vi "Update All Timestamps.vi"(10 "New offset (ns)":i64, 11 "Bytes in":u8[](array[numeric])) -> (2 "Records":i32, 3 "Bytes out":u8[](array[numeric]))   [LabVIEW 2021, in "pcap_Parse_Build_CIF.lvclass"]
doc: "Update all timestamps in the pcap bytestream. This will automatically detect if a global header is present and will work on both full pcap streams to/from disk and pcap packets to/from FIFO. If no global header is found it will default to CIF channel format (little endian, ns timestamp)."
uses:
  pcap_Parse_Build_CIF.lvclass
  pcap_Parse_Build_CIF.lvclass/pcap_Parse_Build_CIF.ctl
  Add Error.vi
  <vilib>/CIF Foundation/CIF Utilities/DataTypes/Flatten Unflatten/Unflatten U32.vi
  Build/SubVIs/Flatten Packet Header.vi
  <vilib>/CIF Foundation/CIF Utilities/DataTypes/Flatten Unflatten/Flatten U32.vi
  Add Error Core.vi
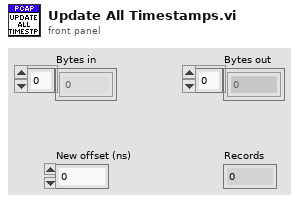
[diagram p1: front panel]
types:
  T1 = typedef "pcap_Parse_Build_CIF.lvclass/Packet Header.ctl" = cluster{"Timestamp (s)":u32, "Timestamp (ns)":u32, "Inc Length":u32, "Orig Length":u32}
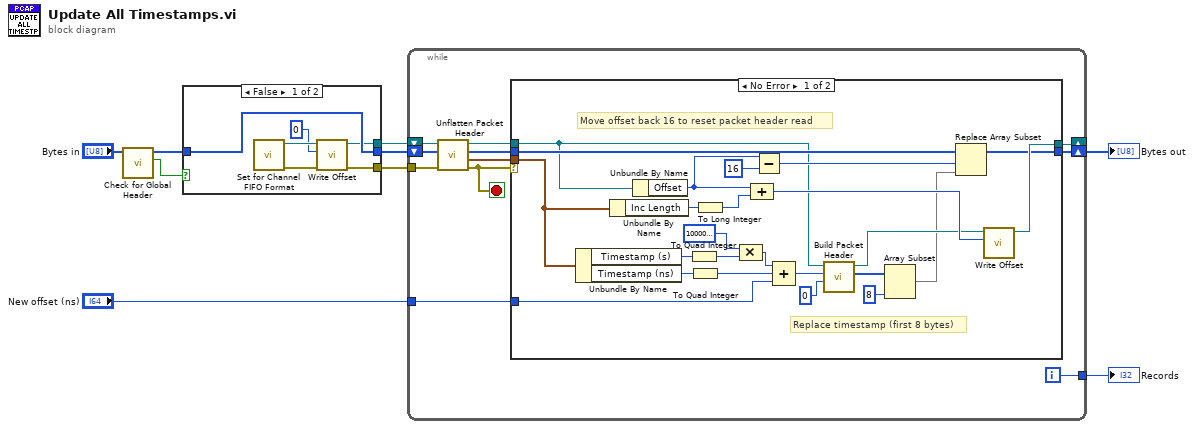
[diagram p0: block diagram]
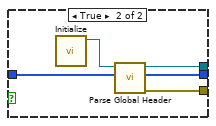
[diagram p3: hidden frame]
diagram:
  n1 = call "Check for Global Header.vi"("Bytes in"="Bytes in") -> ("Global Header Present"=w9:bool, "Bytes out"=w6:u8[])  [unwired: 8 in, 1 out]
  n2 = case shown="False" w9 {
    tunnel: [w11 w16] -> w5
    tunnel: w6 -> [w13 w19]
    tunnel: [w13 w18] -> w8
    tunnel: [w14 w17] -> w7
    frame False {
      n3 = call "Set for Channel FIFO Format.vi"() -> ("error out"=w14:errorcluster, "pcap_Parse_Build_CIF out"=w12:refnum<class "pcap_Parse_Build_CIF.lvclass">)  [unwired: 10 in]
      n4 = call "Write Offset.vi"("Offset"=0, "pcap Parse and Build in"=w12) -> ("pcap Parse and Build out"=w11:refnum<class "pcap_Parse_Build_CIF.lvclass">)  [unwired: 8 in, 1 out]
    }
    frame True {
      n5 = call "Initialize.vi"() -> ("pcap Parse and Build out"=w15:refnum<class "pcap_Parse_Build_CIF.lvclass">)  [unwired: 11 in]
      n6 = call "Parse Global Header.vi"("Bytes in"=w19, "pcap Parse and Build in"=w15) -> ("error out"=w17:errorcluster, "Bytes out"=w18:u8[], "pcap Parse and Build out"=w16:refnum<class "pcap_Parse_Build_CIF.lvclass">)  [unwired: 6 in, 1 out]
    }
  }
  n7 = while {
    tunnel: w7 -> [w29]
    shift-right: [w27] -> _
    shift-left: w5 -> [w28]
    shift-right: [w22] -> w3
    shift-left: w8 -> [w30]
    tunnel: "New offset (ns)" -> [w25]
    tunnel: [w20] -> w1
    i -> [w20]
    stop <- w21 stop-if-true
    n8 = call "Unflatten Packet Header.vi"("error in (no error)"=w29, "Bytes in"=w30, "pcap Parse and Build in"=w28) -> ("error out"=w21:errorcluster, "Packet Header"=w26:T1, "Bytes out"=w23:u8[], "pcap Parse and Build out"=w24:refnum<class "pcap_Parse_Build_CIF.lvclass">)  [unwired: 5 in]
    n9 = case shown="No Error" w21 {
      tunnel: [w54 w56] -> w27
      tunnel: w26 -> [w52 _]
      tunnel: w25 -> [w50 _]
      tunnel: w24 -> [w35 w56]
      tunnel: w23 -> [w40 w55]
      tunnel: [w38 w55] -> w22
      frame No Error {
        # "Replace timestamp (first 8 bytes)"
        # "Move offset back 16 to reset packet header read"
        n10 = Unbundle By Name(w52) -> ("Timestamp (s)"=w47:u32, "Timestamp (ns)"=w46:u32)
        n11 = Unbundle By Name(w52) -> ("Inc Length"=w48:u32)
        n12 = Unbundle By Name(w35) -> ("Offset"=w41:i32)
        n13 = To Quad Integer(1:w47) -> (0:w45:i64)
        n14 = To Quad Integer(1:w46) -> (0:w43:i64)
        n15 = To Long Integer(number=w48) -> (32bit integer=w36:i32)
        n16 = Compound Arithmetic op=MULTIPLY(i64 1000000000 ("x"), w45) -> (w42:i64)
        n17 = Compound Arithmetic op=ADD(w41, w36) -> (w53:i32)
        n18 = Subtract(x=w41, y=16) -> (x-y=w39:i32)
        n19 = Compound Arithmetic op=ADD(w42, w43, w50) -> (w49:i64)
        n20 = call "Build Packet Header.vi"("Length"=0, "TAI Time (ns)"=w49, "pcap Parse and Build in"=w35) -> ("Flattened Data out"=w34:u8[], "pcap Parse and Build out"=w37:refnum<class "pcap_Parse_Build_CIF.lvclass">)  [unwired: 7 in]
        n21 = Array Subset(array=w34, length=8) -> (w33:u8[])  [unwired: 1 in]
        n22 = Replace Array Subset(array=w40, new element=w33, index=w39) -> (w38:u8[])
        n23 = call "Write Offset.vi"("Offset"=w53, "pcap Parse and Build in"=w37) -> ("pcap Parse and Build out"=w54:refnum<class "pcap_Parse_Build_CIF.lvclass">)  [unwired: 8 in, 1 out]
      }
      frame Error {
      }
    }
  }
  "Bytes out" <- w3
  "Records" <- w1
